vi "Open.vi"   [LabVIEW 2021, in "LMH-Xbox-One-Controller.lvlib"]
uses:
  <instrlib>/Xbox-One-Controller/LMH-Xbox-One-Controller.lvlib
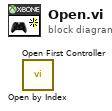
[diagram p0: block diagram]
diagram:
  n1 = call <instrlib>:"Open by Index.vi"() -> ()  [unwired: 9 in, 3 out]
  n2 = call <instrlib>:"Open First Controller.vi"() -> ()  [unwired: 9 in, 3 out]
